vi "Read Any Poly.vi"   [LabVIEW 2018]
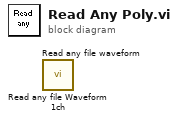
[diagram p0: block diagram]
diagram:
  n1 = call "Read any file Waveform 1ch.vi"() -> ()  [unwired: 7 in, 5 out]
  n2 = call "Read any file waveform.vi"() -> ()  [unwired: 7 in, 5 out]
